vi "Initialise.vi"(6 "Fill Colour":u32(colorbox), 11 "Screen Dimensions":T1) -> (3 "Pixel Data out":u32[][](array[numeric]))   [LabVIEW 2020, in "Raster.lvlib"]
uses:
  Raster.lvlib
  Screen Dimensions.ctl
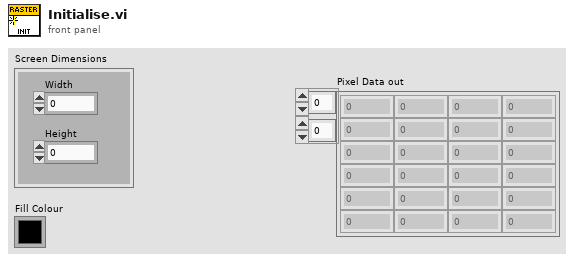
[diagram p1: front panel]
types:
  T1 = typedef "Raster.lvlib/Screen Dimensions.ctl" = cluster{"Width":u32, "Height":u32}
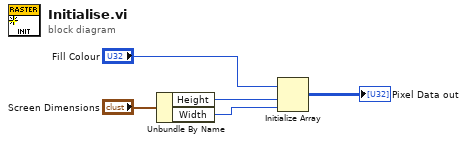
[diagram p0: block diagram]
diagram:
  n1 = Unbundle By Name("Screen Dimensions") -> ("Height"=w1:u32, "Width"=w2:u32)
  n2 = Initialize Array("Fill Colour", w1, w2) -> (→"Pixel Data out":u32[][])
